vi "Config Ext Sensor Scaling.vi"(0 "VISA resource name":refnum<visa-resource-name>, 5 "Element (0: All)":u16(ring) items=["ALL", "Element1", "Element2", "Element3"], 7 "Factor (50.00)":dbl=50.0 min=0.001 max=9999.0 step=0.001 format="%^.3e", 11 "error in (no error)":errorcluster) -> (4 "VISA resource name out":refnum<visa-resource-name>, 15 "error out":errorcluster)   [LabVIEW 2016, in "Yokogawa WT200 Series.lvlib"]
doc: "This VI sends the external sensor scaling command to the WT200 Series."
uses:
  Yokogawa WT200 Series.lvlib
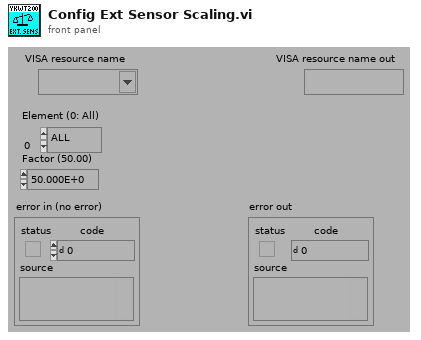
[diagram p1: front panel]
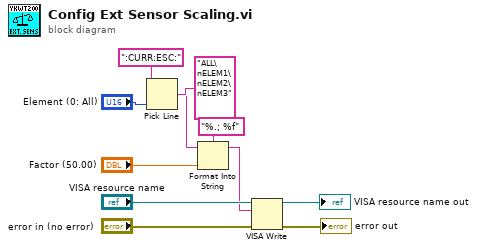
[diagram p0: block diagram]
diagram:
  n1 = Pick Line(string ("")=":CURR:ESC:", multi-line string="ALL\nELEM1\nELEM2\nELEM3", line index="Element (0: All)") -> (output string=w2:string)
  n2 = Format Into String(format string="%.; %f", initial string=w2, "Factor (50.00)") -> (resulting string=w5:string)  [unwired: 1 in, 1 out]
  n3 = VISA Write(VISA resource name="VISA resource name", write buffer=w5, error in (no error)="error in (no error)") -> (VISA resource name out=→"VISA resource name out":refnum<visa-resource-name>, error out=→"error out":errorcluster)  [unwired: 1 out]
